vi "Check Subscription Policy.vi"(9 "Value Changed?":bool, 10 "Topic Value":variant, 11 "SubscriptionPolicy in":refnum<class "SubscriptionPolicy.lvclass">) -> (1 "Boot Subscriber On Transport Failure?":bool, 2 "Notify Subscriber?":bool, 3 "SubscriptionPolicy out":refnum<class "SubscriptionPolicy.lvclass">)   [LabVIEW 2015, in "IMediator.lvlib" / "SubscriptionPolicy.lvclass"]
doc: "<License>\nCopyright © 2017 Composed Systems, LLC | All rights reserved\nwww.composed.io\n\nAuthor: Ethan Stern <ethan.stern@composed.io>\n\nThis software is provided \"AS IS\" WITHOUT WARRANTIES, either express or implied, AND IS FOR EDUCATIONAL PURPOSES ONLY.\n</License>"
uses:
  SubscriptionPolicy.lvclass
  SubscriptionPolicy.lvclass/SubscriptionPolicy.ctl
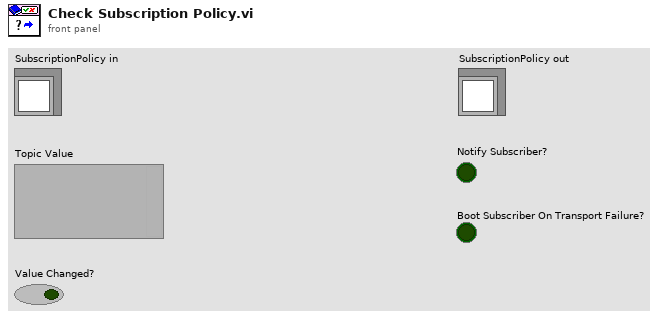
[diagram p1: front panel]
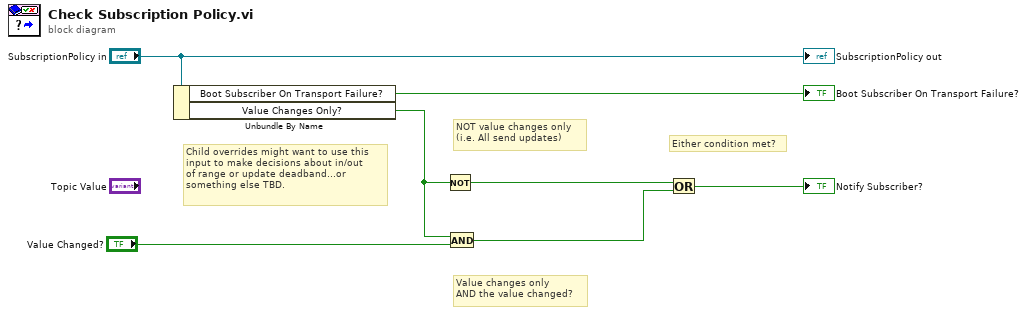
[diagram p0: block diagram]
diagram:
  # "Either condition met?"
  # "Value changes only\nAND the value changed?"
  # "NOT value changes only\n(i.e. All send updates)"
  # "Child overrides might want to use this\ninput to make decisions about in/out\nof range or update deadband...or\nsomething else TBD."
  n1 = Unbundle By Name("SubscriptionPolicy in") -> ("Boot Subscriber On Transport Failure?"=→"Boot Subscriber On Transport Failure?":bool, "Value Changes Only?"=w2:bool)
  n2 = Not ("NOT ValChg Only")(x=w2) -> (.not. x?=w1:bool)
  n3 = And ("ValChg Only AND Val Changed?")(x=w2, y="Value Changed?") -> (x .and. y?=w4:bool)
  n4 = Or ("Notify?")(x=w1, y=w4) -> (x .or. y?=→"Notify Subscriber?":bool)
  "SubscriptionPolicy out" <- "SubscriptionPolicy in"
